vi "Read Min-Max.vi"(0 "VISA resource name":refnum<visa-resource-name>, 7 "Input (0: A)":u16(ring) items=["A", "B"], 11 "error in (no error)":errorcluster) -> (4 "VISA resource name out":refnum<visa-resource-name>, 8 "Min Value":dbl min=-1500.0 max=300000.0 step=0.0001 format="%^.4e", 10 "Max Value":dbl min=-1500.0 max=300000.0 step=0.0001 format="%^.4e", 15 "error out":errorcluster)   [LabVIEW 2013, in "Lake Shore Cryotronics 331.lvlib"]
doc: "This VI querys the instrument for an inputs min/max readings."
uses:
  Lake Shore Cryotronics 331.lvlib
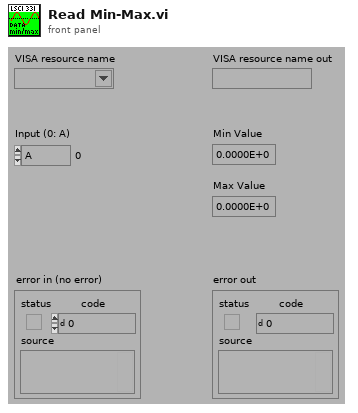
[diagram p1: front panel]
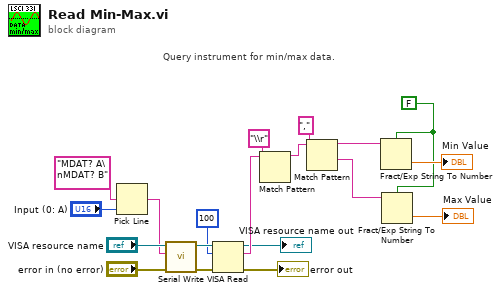
[diagram p0: block diagram]
diagram:
  w4 = FALSE ("use system decimal point (T)")
  # "Query instrument for min/max data."
  n1 = Pick Line(multi-line string="MDAT? A\nMDAT? B", line index="Input (0: A)") -> (output string=w1:string)  [unwired: 1 in]
  n2 = call "Serial Write.vi"("error in (no error)"="error in (no error)", "Write Buffer (\"\")"=w1, "VISA resource name"="VISA resource name") -> ("error out"=w16:errorcluster, "VISA resource name out"=w17:refnum<visa-resource-name>)  [unwired: 6 in, 1 out]
  n3 = VISA Read(VISA resource name=w17, byte count=100, error in (no error)=w16) -> (VISA resource name out=→"VISA resource name out":refnum<visa-resource-name>, read buffer=w14:string, error out=→"error out":errorcluster)  [unwired: 1 out]
  n4 = Match Pattern(string=w14, regular expression="\\r") -> (before substring=w11:string)  [unwired: 1 in, 3 out]
  n5 = Match Pattern(string=w11, regular expression=",") -> (before substring=w10:string, after substring=w9:string)  [unwired: 1 in, 2 out]
  n6 = Fract/Exp String To Number(use system decimal point (T)=w4, string=w10) -> (number=→"Min Value":dbl)  [unwired: 2 in, 1 out]
  n7 = Fract/Exp String To Number(use system decimal point (T)=w4, string=w9) -> (number=→"Max Value":dbl)  [unwired: 2 in, 1 out]
